vi "ColorizeREPL.vi"(0 "refs":cluster{"Code":refnum<vi>, "Panel":refnum<vi>}, 4 "Add Spaces?":bool) -> (8 "Value":string)   [LabVIEW 2016]
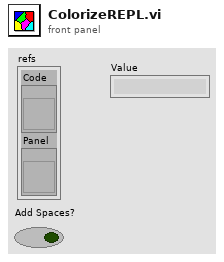
[diagram p1: front panel]
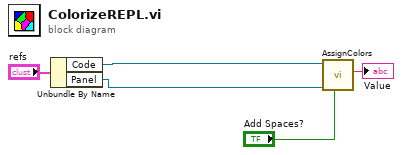
[diagram p0: block diagram]
diagram:
  n1 = Unbundle By Name("refs") -> ("Code"=w1:refnum<vi>, "Panel"=w4:refnum<vi>)
  n2 = call "AssignColors.vi"("Add Spaces?"="Add Spaces?", "Front Panel"=w4, "Code"=w1) -> ("Value"=→"Value":string)  [unwired: 8 in]
